vi "Update Attribute Tree.vi"(6 "Panel Refnum In":refnum<vi>, 8 "error in":errorcluster, 9 "Flush Tree?":bool, 10 "Tree Control In":refnum<vi>, 11 "Camera Name In":T1 caption="Session In") -> (0 "error out":errorcluster, 2 "Tree Control Out":refnum<vi>, 3 "Session Out":T1)   [LabVIEW 2023]
doc: "The Update Attribute Tree subVI, enumerates the attributes available for the camera and populates the Attribute Tree control with the attribute list."
uses:
  <vilib>/userdefined/High Color/IMAQdx.ctl
  <vilib>/vision/driver/NI_Vision_Acquisition_Software.lvlib
  <resource>/objmgr/imaqdx.rc
panel:
  # "Overview: Demonstrates\nRequirements: Vision Acquisition Software\nInstructions: Run the VI"
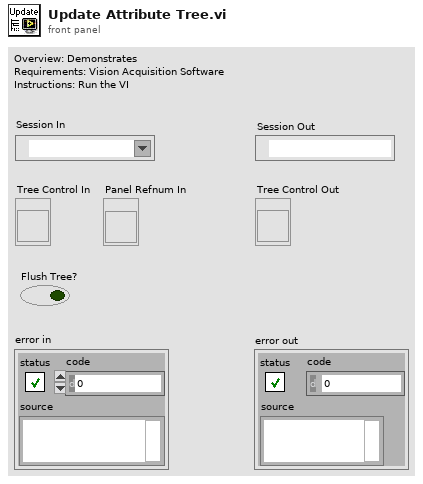
[diagram p1: front panel]
types:
  T1 = typedef "IMAQdx.ctl" = refnum<k21>
  T2 = typedef "NI_Vision_Acquisition_Software.lvlib/IMAQdx Attribute Type.ctl" = enum32{"U32", "I64", "DBL", "String", "Enum", "Bool", "Command"}
  T3 = cluster{"Attribute Type":T2, "Readable":bool, "Writable":bool, "Attribute Name":string}[]
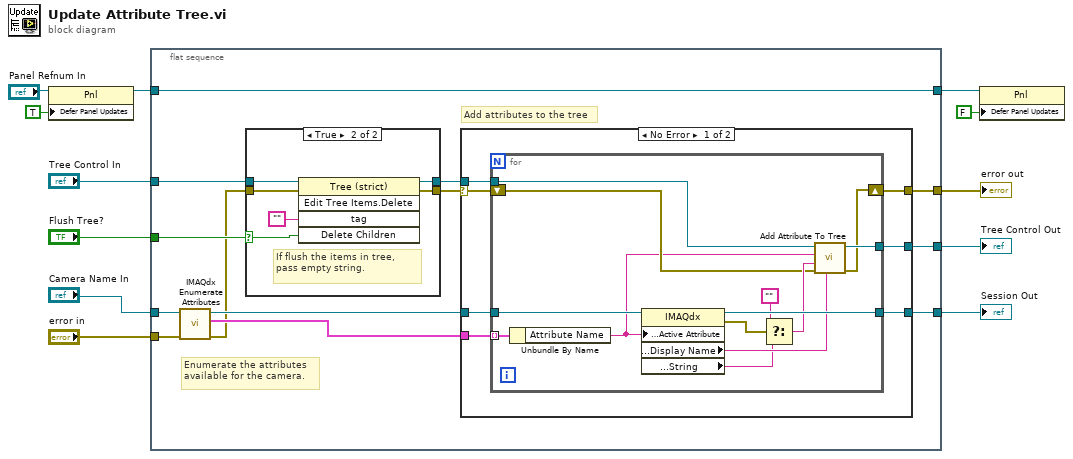
[diagram p0: block diagram]
diagram:
  n1 = property class="Pnl"(reference="Panel Refnum In", "Defer Panel Updates"=TRUE) -> (reference out=w2:refnum<vi>)  [unwired: 1 in, 1 out]
  n2 = flat-sequence {
    tunnel: "Tree Control In" -> [w25]
    tunnel: "Flush Tree?" -> [w24]
    tunnel: "Camera Name In" -> [w23]
    tunnel: "error in" -> [w22]
    tunnel: [w21] -> w7
    tunnel: [w20] -> w6
    tunnel: [w19] -> w5
    tunnel: [w13] -> w1
    tunnel: w2 -> [w13]
    frame #0 {
      # "Add attributes to the tree"
      # "Enumerate the attributes available for the camera."
      n3 = call <vilib>:"IMAQdx Enumerate Attributes.vi"("error in"=w22, "Session In"=w23) -> ("error out"=w14:errorcluster, "Attribute Information Array"=w17:T3, "Session Out"=w18:T1)  [unwired: 2 in, 5 out]
      n4 = case shown="True" w24 {
        selector: w24 -> [_ w28]
        tunnel: [w27 w33] -> w16
        tunnel: [w26 w32] -> w15
        tunnel: w14 -> [w26 w31]
        tunnel: w25 -> [w27 w29]
        frame False {
        }
        frame True {
          # "If flush the items in tree, pass empty string."
          n5 = invoke class="Tree (strict)" method="Edit Tree Items.Delete"(reference=w29, error in=w31, "tag"="", "Delete Children"=w28) -> (reference out=w33:refnum<vi>, error out=w32:errorcluster)  [unwired: 1 in, 3 out]
        }
      }
      n6 = case shown="No Error" w15 {
        selector: w15 -> [w38 w56]
        tunnel: w17 -> [w40 _]
        tunnel: w16 -> [w39 w54]
        tunnel: w18 -> [w37 w55]
        tunnel: [w34 w56] -> w21
        tunnel: [w36 w55] -> w19
        tunnel: [w35 w54] -> w20
        frame No Error {
          n7 = for {
            tunnel: w40 -> [w53] mode=indexing
            tunnel: w39 -> [w50]
            tunnel: w37 -> [w52]
            tunnel: [w51] -> w36
            tunnel: [w45] -> w35
            shift-right: [w41] -> w34
            shift-left: w38 -> [w46]
            n8 = Unbundle By Name(w53) -> ("Attribute Name"=w44:string)
            n9 = property class="IMAQdx"(reference=w52, "Camera Attributes:Active Attribute"=w44) -> (reference out=w51:T1, error out=w49:errorcluster, "Camera Attributes:Display Name"=w43:string, "Camera Attributes:Value:String"=w42:string)  [unwired: 1 in]
            n10 = Select(t="", s=w49, f=w42) -> (s? t:f=w48:string)
            n11 = call "Add Attribute To Tree.vi"("Display Name"=w43, "error in"=w46, "Value"=w48, "Attribute Name"=w44, "Attribute Table In"=w50) -> ("error out"=w41:errorcluster, "Attribute Table Out"=w45:refnum<vi>)  [unwired: 5 out]
          }
        }
        frame Error {
        }
      }
    }
  }
  n12 = property class="Pnl"(reference=w1, "Defer Panel Updates"=FALSE) -> ()  [unwired: 1 in, 2 out]
  "error out" <- w7
  "Session Out" <- w5
  "Tree Control Out" <- w6
